vi "set TIFF resolultion tag via command line.vi"(7 "tiffset.exe file path":path, 8 "y pixels per m":dbl=0.5, 9 "x pixels per m":dbl=0.5, 11 "TIFF file path":path) -> ()   [LabVIEW 2012]
doc: "This VI sets the TIFF tags XResolution and YResolution by calling the command line tool tiffset.exe via the System Exce.vi. This workaround is necessary because libtiff3.dll requires these tags to be handed over as data type RATIONAL, a data type that doesn't exist in LabView. \nThe values represent number of pixels per micrometer. These will be correctly interpreted by ImageJ, but other software may interpret these values incorrectly as number of pixels per centimeter. In those cases values will need to be adjusted by a factor of 1e-6."
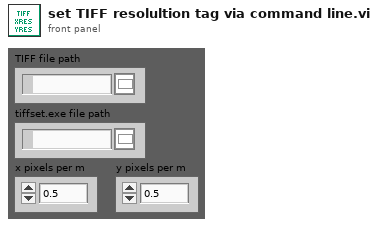
[diagram p1: front panel]
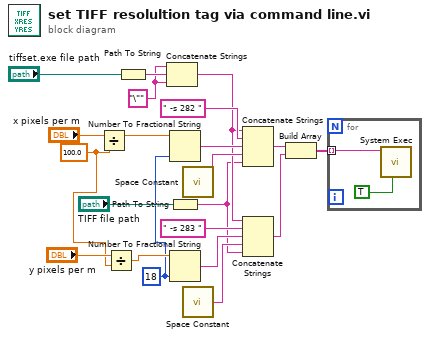
[diagram p0: block diagram]
diagram:
  w1 = i16 18 ("precision (6)")
  w2 = 100.0 ("y")
  w15 = "\"" ("string")
  n1 = Divide(x="x pixels per m", y=w2) -> (x/y=w4:dbl)
  n2 = Divide(x="y pixels per m", y=w2) -> (x/y=w3:dbl)
  n3 = Path To String(path="tiffset.exe file path") -> (string=w16:string)
  n4 = Concatenate Strings(w15, w16, w15) -> (w11:string)
  n5 = Number To Fractional String(number=w4, precision (6)=w1) -> (F-format string=w20:string)  [unwired: 2 in]
  n6 = Path To String(path="TIFF file path") -> (string=w7:string)
  n7 = Number To Fractional String(number=w3, precision (6)=w1) -> (F-format string=w9:string)  [unwired: 2 in]
  n8 = call <vilib>:"Space Constant.vi"() -> ("String"=w21:string)
  n9 = call <vilib>:"Space Constant.vi"() -> ("String"=w8:string)
  n10 = Concatenate Strings(w11, " -s 282 " ("string"), w20, w21, w7) -> (w14:string)
  n11 = Concatenate Strings(w11, " -s 283 " ("string"), w9, w8, w7) -> (w13:string)
  n12 = Build Array(w14, w13) -> (w12:string[])
  n13 = for {
    tunnel: w12 -> [w22] mode=indexing
    n14 = call <vilib>:"System Exec.vi"("run minimized? (F)"=TRUE, "command line"=w22) -> ()  [unwired: 6 in, 4 out]
  }
